vi "MGI Destroy.vi"(8 "error in (no error)":errorcluster) -> (0 "error out":errorcluster)   [LabVIEW 2016, in "MGI Error Reporter Base.lvclass"]
doc: "Stop the Error Reporter daemon from executing if no other VIs are currently using it.\n\n\n\nAuthored by Shawn Walpole\nsupport@mooregoodideas.com\nwww.mooregoodideas.com\n\nCopyright (c) 2013, Moore Good Ideas, Inc.\n\nAll rights reserved.\n\nRedistribution and use in source and binary forms, with or without modification, are permitted provided that the following conditions are met:\n\n * Redistributions of source code must retain the above copyright notice, this list of conditions and the following disclaimer.\n * Redistributions in binary form must reproduce the above copyright notice, this list of conditions and the following disclaimer in the documentation and/or other materials provided with the distribution.\n * Neither the name of Moore Good Ideas, Inc. nor the names of its contributors may be used to endorse or promote products derived from this software without specific prior written permission.\n\nTHIS SOFTWARE IS PROVIDED BY THE COPYRIGHT HOLDERS AND CONTRIBUTORS \"AS IS\" AND ANY EXPRESS OR IMPLIED WARRANTIES, INCLUDING, BUT NOT LIMITED TO, THE IMPLIED WARRANTIES OF MERCHANTABILITY AND FITNESS FOR A PARTICULAR PURPOSE ARE DISCLAIMED. IN NO EVENT SHALL THE COPYRIGHT OWNER OR CONTRIBUTORS BE LIABLE FOR ANY DIRECT, INDIRECT, INCIDENTAL, SPECIAL, EXEMPLARY, OR CONSEQUENTIAL DAMAGES (INCLUDING, BUT NOT LIMITED TO, PROCUREMENT OF SUBSTITUTE GOODS OR SERVICES; LOSS OF USE, DATA, OR PROFITS; OR BUSINESS INTERRUPTION) HOWEVER CAUSED AND ON ANY THEORY OF LIABILITY, WHETHER IN CONTRACT, STRICT LIABILITY, OR TORT (INCLUDING NEGLIGENCE OR OTHERWISE) ARISING IN ANY WAY OUT OF THE USE OF THIS SOFTWARE, EVEN IF ADVISED OF THE POSSIBILITY OF SUCH DAMAGE."
uses:
  <userlib>/_MGI/Error Reporter/MGI Error Reporter Base/MGI Error Reporter Base.lvclass
  <userlib>/_MGI/Error Reporter/MGI Error Reporter Base/Protected/MGI Cmd Enum.ctl
  <userlib>/_MGI/Error Reporter/MGI Error Reporter Base/Private/MGI Globals.vi
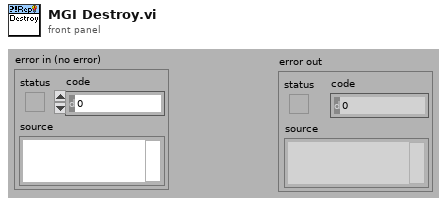
[diagram p1: front panel]
types:
  T1 = typedef "MGI Error Reporter Base.lvclass/MGI Cmd Enum.ctl" = enum16{"Quit", "Show UI"}
  T2 = enum32{"Bad", "Idle", "Run top level", "Running"}[]
  T3 = enum32{"Bad", "Idle", "Run top level", "Running"}
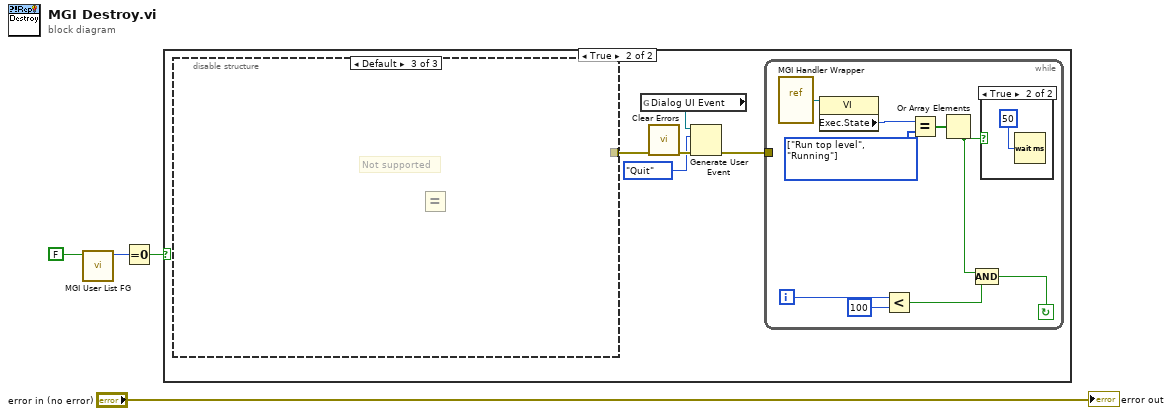
[diagram p0: block diagram]
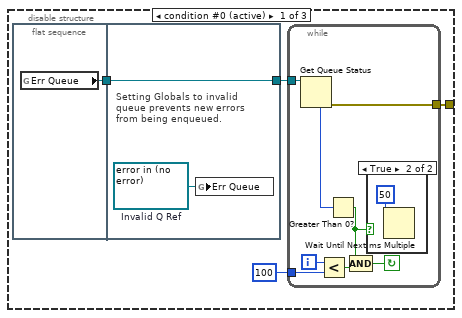
[diagram p3: hidden frame]
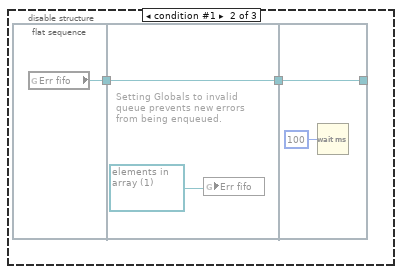
[diagram p5: hidden frame]
diagram:
  n1 = call <userlib>:"MGI User List FG.vi"("Create? (F:Destroy)"=FALSE) -> ("# Top Level Users"=w4:i32)  [unwired: 10 out]
  n2 = Equal To 0?(x=w4) -> (x = 0?=w3:bool)
  n3 = case shown="True" w3 {
    frame False {
    }
    frame True {
      n4 = disable-structure shown="Default" {
        disable-tunnel: [w12 _ _] -> w7
        frame condition #0 (active) {
          n5 = flat-sequence {
            tunnel: [w23] -> w13
            tunnel: w13 -> [w25]
            tunnel: [w25] -> w11
            frame #0 {
              n6 = global read "MGI Globals.vi" "Err Queue"() -> (w23:refnum<queue>)
            }
            frame #1 {
              w24 = refnum<queue> refnum  # Invalid Q Ref
              # "Setting Globals to invalid queue prevents new errors from being enqueued."
              n7 = global write "MGI Globals.vi" "Err Queue"(w24) -> ()
            }
          }
          n8 = while {
            tunnel: w11 -> [w21]
            tunnel: [w16] -> w12
            tunnel: 100 ("y") -> [w14]
            i -> [w18]
            stop <- w19 continue-if-true
            n9 = Get Queue Status(queue=w21) -> (error out=w16:errorcluster, # elements in queue=w20:i32)  [unwired: 1 in, 7 out]
            n10 = Less?(x=w18, y=w14) -> (x < y?=w17:bool)
            n11 = Greater Than 0?(x=w20) -> (x > 0?=w15:bool)
            n12 = Compound Arithmetic op=AND(w15, w17) -> (w19:bool)
            n13 = case shown="True" w15 {
              frame False {
              }
              frame True {
                n14 = Wait Until Next ms Multiple(millisecond multiple=u32 50) -> ()  [unwired: 1 out]
              }
            }
          }
        }
        frame condition #1 {
          n15 = flat-sequence {
            tunnel: [w28] -> w27
            tunnel: w27 -> [w30]
            tunnel: [w30] -> w26
            tunnel: [w32] -> _
            tunnel: w26 -> [w32]
            frame #0 {
              n16 = global read "MGI Globals.vi" "Err fifo"() -> (w28:refnum<k33>)
            }
            frame #1 {
              # "Setting Globals to invalid queue prevents new errors from being enqueued."
              n17 = global write "MGI Globals.vi" "Err fifo"(refnum<k33> refnum ("Err fifo")) -> ()
            }
            frame #2 {
              n18 = Wait (ms)(milliseconds to wait=u32 100) -> ()  [unwired: 1 out]
            }
          }
        }
        frame condition #2 {
          # "Not supported"
          n19 = Equal?() -> ()  [unwired: 2 in, 1 out]
        }
      }
      n20 = global read "MGI Globals.vi" "Dialog UI Event"() -> (w5:refnum<user-event>)
      n21 = call <vilib>:"Clear Errors.vi"("error in (no error)"=w7) -> ("error out"=w9:errorcluster)  [unwired: 1 in, 5 out]
      n22 = Generate User Event(user event=w5, event data cluster=MGI_Cmd_Enum."Quit" ("event data"), error in=w9) -> (error out=w6:errorcluster)  [unwired: 1 in, 1 out]
      n23 = while {
        tunnel: w6 -> [_]
        i -> [w37]
        stop <- w35 continue-if-true
        w39 = T2 [enum."Run top level", enum."Running"] items=["Bad", "Idle", "Run top level", "Running"]
        n24 = vi-ref <userlib>:"MGI Handler Wrapper.vi"() -> (w41:refnum<vi>)
        n25 = property class="VI"(reference=w41) -> ("Exec.State"=w40:T3)  [unwired: 1 in, 2 out]
        n26 = Less?(x=w37, y=100) -> (x < y?=w36:bool)
        n27 = Equal?(x=w40, y=w39) -> (x = y?=w38:bool[])
        n28 = Or Array Elements(Boolean array=w38) -> (logical OR=w33:bool)
        n29 = Compound Arithmetic op=AND(w33, w36) -> (w35:bool)
        n30 = case shown="True" w33 {
          frame False {
          }
          frame True {
            n31 = Wait (ms)(milliseconds to wait=u32 50) -> ()  [unwired: 1 out]
          }
        }
      }
    }
  }
  "error out" <- "error in (no error)"
